vi "CheckInLogic.vi"(0 "all rows in":string[][](array[string]), 1 "Student ID":i32, 2 "Flag":T1=enum."Seconds", 3 "Check In":T1=enum."Seconds", 4 "date/time string":string, 5 "Time Cluster":T2) -> (14 "all rows out":string[][](array[string]))   [LabVIEW 2013]
uses:
  Controls/SpreadsheetColumns.ctl
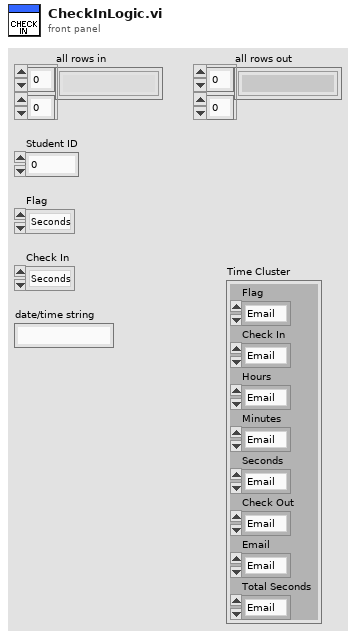
[diagram p1: front panel]
types:
  T1 = typedef "SpreadsheetColumns.ctl" = enum16{"Email", "CheckIn", "CheckOut", "Flag", "Hours", "Minutes", "Seconds", "Total Seconds", "Cat Points"}
  T2 = cluster{"Flag":T1, "Check In":T1, "Hours":T1, "Minutes":T1, "Seconds":T1, "Check Out":T1, "Email":T1, "Total Seconds":T1}
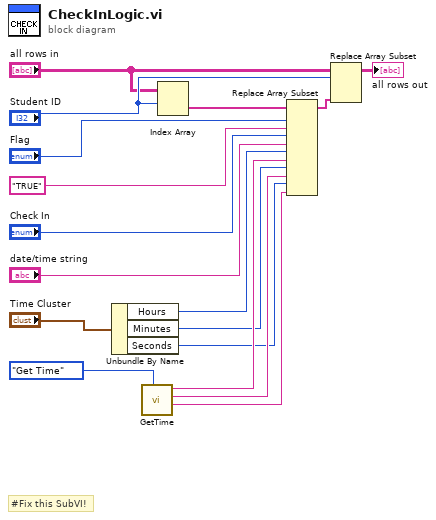
[diagram p0: block diagram]
diagram:
  # "#Fix this SubVI!"
  n1 = Unbundle By Name("Time Cluster") -> ("Hours"=w10:T1, "Minutes"=w11:T1, "Seconds"=w12:T1)
  n2 = call "GetTime.vi"("State"=enum16{"Get Time", "Calculate Differential"}."Get Time") -> ("Seconds"=w15:string, "Minutes"=w14:string, "Hours"=w13:string)  [unwired: 5 in, 3 out]
  n3 = Index Array(array="all rows in", index (row)="Student ID") -> (element=w9:string[])  [unwired: 1 in]
  n4 = Replace Array Subset(array=w9, new element #1="TRUE" ("new element/subarray"), index #1="Flag", new element #2="date/time string", index #2="Check In", new element #3=w13, index #3=w10, new element #4=w14, index #4=w11, new element #5=w15, index #5=w12) -> (w16:string[])
  n5 = Replace Array Subset(array="all rows in", new element=w16, index (row)="Student ID") -> (→"all rows out":string[][])  [unwired: 1 in]
